vi "Texte aus Ring herausholen.vi"(8 "Def.CalGas":refnum<vi>, 9 "Gas":i32, 10 "Element Messbereich":i32, 11 "Element Einheit":i32) -> (2 "Messberich":T1, 3 "Einheit":T1)   [LabVIEW 2020, in "CalGas Aufschaltung.lvlib"]
uses:
  CalGas Aufschaltung.lvlib
  Visualisierungs Elemente/String - Ausgabefeld.ctl
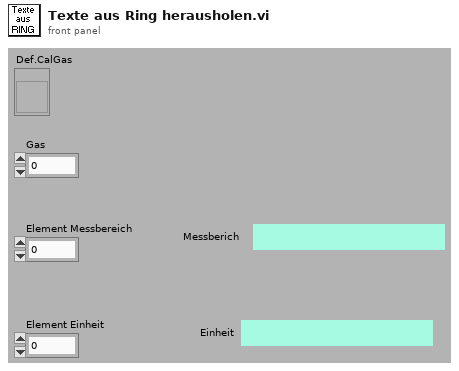
[diagram p1: front panel]
types:
  T1 = typedef "String - Ausgabefeld.ctl" = string
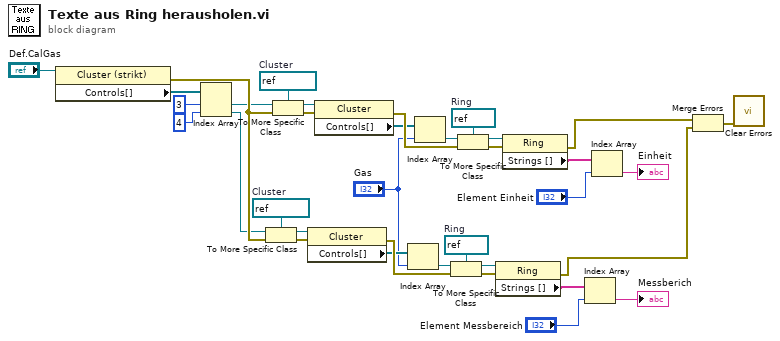
[diagram p0: block diagram]
diagram:
  w15 = refnum<vi> refnum  # Ring
  w12 = refnum<vi> refnum  # Cluster
  w26 = refnum<vi> refnum  # Ring
  w31 = refnum<vi> refnum  # Cluster
  n1 = property class="Cluster (strikt)"(reference="Def.CalGas") -> (error out=w33:errorcluster, "Controls[]"=w28:refnum<vi>[])  [unwired: 1 in, 1 out]
  n2 = Index Array(array=w28, index #1=3 ("Index"), index #2=4 ("Index")) -> (element #1=w29:refnum<vi>, element #2=w11:refnum<vi>)
  n3 = To More Specific Class(target class=w12, reference=w11, error in=w33) -> (specific class reference=w13:refnum<vi>, error out=w5:errorcluster)
  n4 = To More Specific Class(target class=w31, reference=w29, error in=w33) -> (specific class reference=w30:refnum<vi>, error out=w7:errorcluster)
  n5 = property class="Cluster"(reference=w13, error in=w5) -> (error out=w35:errorcluster, "Controls[]"=w14:refnum<vi>[])  [unwired: 1 out]
  n6 = property class="Cluster"(reference=w30, error in=w7) -> (error out=w34:errorcluster, "Controls[]"=w27:refnum<vi>[])  [unwired: 1 out]
  n7 = Index Array(array=w14, index="Gas") -> (element=w17:refnum<vi>)
  n8 = Index Array(array=w27, index="Gas") -> (element=w24:refnum<vi>)
  n9 = To More Specific Class(target class=w15, reference=w17, error in=w35) -> (specific class reference=w16:refnum<vi>, error out=w4:errorcluster)
  n10 = To More Specific Class(target class=w26, reference=w24, error in=w34) -> (specific class reference=w25:refnum<vi>, error out=w6:errorcluster)
  n11 = property class="Ring"(reference=w16, error in=w4) -> (error out=w2:errorcluster, "Strings []"=w18:string[])  [unwired: 1 out]
  n12 = property class="Ring"(reference=w25, error in=w6) -> (error out=w1:errorcluster, "Strings []"=w23:string[])  [unwired: 1 out]
  n13 = Index Array(array=w18, index="Element Messbereich") -> (element=→"Messberich":string)
  n14 = Index Array(array=w23, index="Element Einheit") -> (element=→"Einheit":string)
  n15 = Merge Errors(w1, w2) -> (w3:errorcluster)
  n16 = call <vilib>:"Clear Errors.vi"("error in (no error)"=w3) -> ()  [unwired: 5 in, 2 out]
